vi "HostIndex_Read.vi"(0 "Axis In":T1, 11 "error in (no error)":errorcluster) -> (4 "Axis Out":T1, 6 "Index":T2, 15 "error out":errorcluster)   [LabVIEW 2009]
doc: "Set Host Index parameter."
uses:
  typedefs/Ultra3000/Cmds.ctl
  typedefs/Ultra3000/Func.ctl
  typedefs/Ultra3000/Index_Numeric.ctl
  typedefs/AxisSelect_Enum.ctl
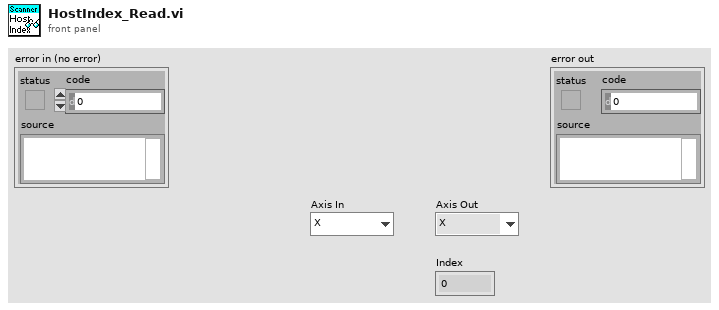
[diagram p1: front panel]
types:
  T1 = typedef "AxisSelect_Enum.ctl" = enum16{"X", "Y", "Z", "Axis Space"}
  T2 = typedef "Index_Numeric.ctl" = u8
  T3 = typedef "Func.ctl" = u16
  T4 = typedef "Cmds.ctl" = u16
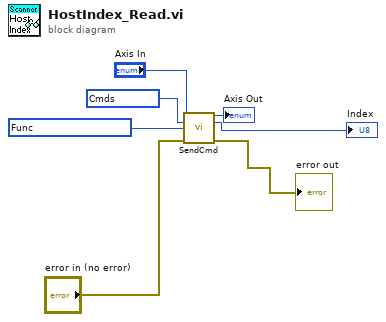
[diagram p0: block diagram]
diagram:
  w5 = T3 ? items=["Read Working Value", "Write Working Value", "Read Non-Volatile Value", "Write Non-Volatile and Woring Value", "Copy Non-Volatile Value to Working Value", "Copy Working Value to Non-Volatile Value", "Read Default Value", "Copy Default Value to Non-Volatile and Working Values", "Read Min Value", "Read Max Value", "Read Array Index Min", "Read Array Index Max"] ("Function")
  w6 = T4 ? items=["Position Command", "Run Status", "Fault Status", "Position Error", "Auto-Start Homing", "Start Homing", "Homing Type", "Motor Position", "Velocity Motor", "Power-Up Status", "Drive Name", "Position Window Size", "Position Window Time", "Zero Speed Limit", "Speed Window Size", "Up to Speed Limit", "Forward Current Limit", "Reverse Current Limit", "Override Mode", "Operation Mode", "Host Control Mode", "Reset Drive", "Drive Enable", "Setpoint Current", "Setpoint Velocity", "Setpoint Acceleration", "Reset Faults", "Position Comparator", "Postition Comparator Polarity", "Position Rollover Enable", "Baud Rate", "Frame Format", "Drive Address", "Broadcast Address", "Auto-start Indexing", "Start Index", "Host Index", "Index Type", "Index Dist/Pos", "Index Reg Dist", "Index Velocity", "Index Acceleration", "Index Deceleration", "Index Dwell", "Index Count", "Index Termination", "Index Pointer", "Index Abort Deceleration", "Positive Soft Pos Limit", "Define Home", "Negative Soft Pos Limit"] ("Command")
  n1 = call "SendCmd.vi"("Axis In"="Axis In", "Command"=w6, "Function"=w5, "error in (no error)"="error in (no error)") -> ("Axis Out"=→"Axis Out":T1, "Data"=→"Index":i32, "error out"=→"error out":errorcluster)  [unwired: 8 in, 1 out]
